vi "SParam Configure Measurement.vi"(8 "error in":errorcluster, 10 "Test Configuration":T2={"Action"=enum."Measure", "Power Level (dBm)"=0.0, "External Gain (dB)"=0.0, "Frequency Sweep"={"Start Frequency (Hz)"=4000000000.0, "Stop Frequency (Hz)"=26000000000.0, "Step Size (Hz)"=200.0}, "Type of Stimulus"=enum."CW", "Pulse Width (s)"=0.0, "PRI (s)"=0.0, "IF Bandwidth (Hz)"=0.0, "Average Mode"=enum."Per Sweep", "Number of Averages"=0, "SnP File Path"=path "", "Calibration File Path"=path ""} {"Frequency Sweep"."Step Size (Hz)" format="%#_6p"; "Frequency Sweep"."Stop Frequency (Hz)" format="%.3p"; "Frequency Sweep"."Start Frequency (Hz)" format="%.3p"}, 11 "S-Par Reference In":T1) -> (0 "error out":errorcluster, 3 "S-Par Reference Out":T1)   [LabVIEW 2023]
uses:
  <vilib>/niSPML/Typedefs/Session Handle.ctl
  <vilib>/niSPML/S-Par Reference.lvclass
  Controls/Test Config - SParam_VST.ctl
  <vilib>/niSPML/S-Parameter Measurements.lvlib
  <vilib>/niSPML/Configure Stimulus (CW).vi
  <vilib>/niSPML/Configure Stimulus (Pulsed CW).vi
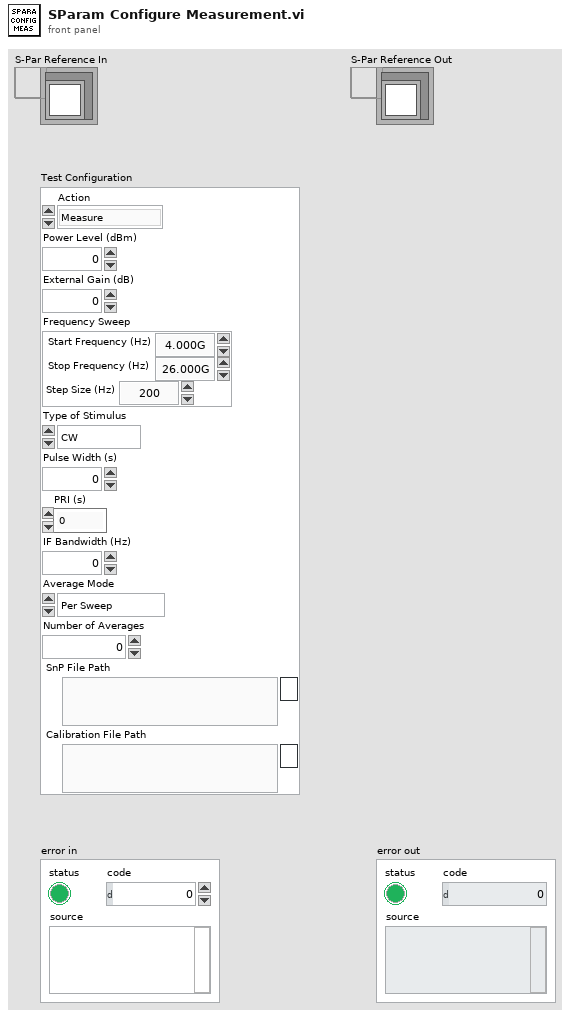
[diagram p1: front panel]
types:
  T1 = typedef "S-Parameter Measurements.lvlib/S-Par Reference.lvclass/Session Handle.ctl" = refnum<data-value>
  T2 = typedef "Test Config - SParam_VST.ctl" = cluster{"Action":enum32{"Calibrate", "Measure"}, "Power Level (dBm)":dbl, "External Gain (dB)":dbl, "Frequency Sweep":cluster{"Start Frequency (Hz)":dbl, "Stop Frequency (Hz)":dbl, "Step Size (Hz)":dbl}, "Type of Stimulus":enum16{"CW", "Pulsed CW"}, "Pulse Width (s)":dbl, "PRI (s)":dbl, "IF Bandwidth (Hz)":dbl, "Average Mode":enum16{"Per Sweep", "Per Point"}, "Number of Averages":i32, "SnP File Path":path, "Calibration File Path":path}
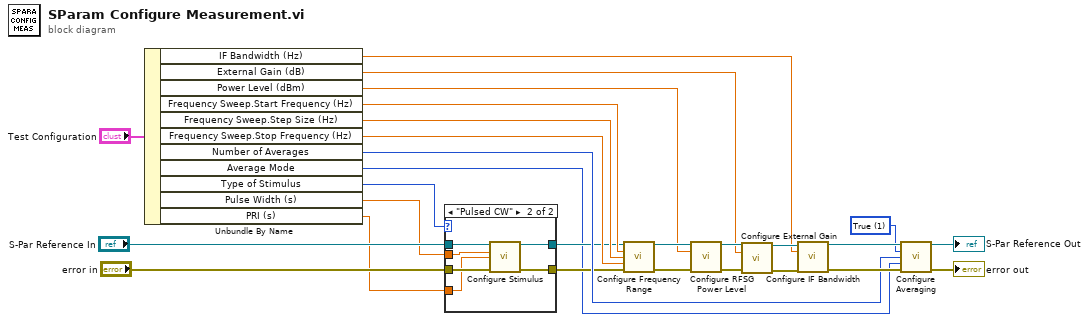
[diagram p0: block diagram]
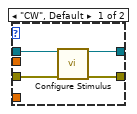
[diagram p2: hidden frame]
diagram:
  w19 = 1 items=["False", "True"] ("Averaging Enabled")
  n1 = Unbundle By Name("Test Configuration") -> ("IF Bandwidth (Hz)"=w12:dbl, "External Gain (dB)"=w13:dbl, "Power Level (dBm)"=w14:dbl, "Frequency Sweep.Start Frequency (Hz)"=w17:dbl, "Frequency Sweep.Step Size (Hz)"=w16:dbl, "Frequency Sweep.Stop Frequency (Hz)"=w15:dbl, "Number of Averages"=w11:i32, "Average Mode"=w1:enum16{"Per Sweep", "Per Point"}, "Type of Stimulus"=w8:enum16{"CW", "Pulsed CW"}, "Pulse Width (s)"=w3:dbl, "PRI (s)"=w2:dbl)
  n2 = case shown="\"Pulsed CW\"" w8 {
    tunnel: "S-Par Reference In" -> [w31 w37]
    tunnel: [w30 w36] -> w6
    tunnel: "error in" -> [w29 w35]
    tunnel: [w28 w34] -> w4
    tunnel: w3 -> [_ w33]
    tunnel: w2 -> [_ w32]
    frame "CW", Default {
      n3 = call-poly <vilib>:"Configure Stimulus.vi"("S-Par Reference In"=w31, "error in"=w29) -> ("S-Par Reference Out"=w30:T1, "error out"=w28:errorcluster)  [unwired: 12 in]
    }
    frame "Pulsed CW" {
      n4 = call-poly <vilib>:"Configure Stimulus.vi"("S-Par Reference In"=w37, "Pulse Width (s)"=w33, "PRI (s)"=w32, "error in"=w35) -> ("S-Par Reference Out"=w36:T1, "error out"=w34:errorcluster)  [unwired: 10 in]
    }
  }
  n5 = call <vilib>:"Configure Frequency Range.vi"("S-Par Reference In"=w6, "Start Frequency (Hz)"=w17, "Frequency Step (Hz)"=w16, "Stop Frequency (Hz)"=w15, "error in"=w4) -> ("S-Par Reference Out"=w21:T1, "error out"=w20:errorcluster)  [unwired: 9 in]
  n6 = call <vilib>:"Configure RFSG Power Level.vi"("S-Par Reference In"=w21, "Power Level (dBm)"=w14, "error in"=w20) -> ("S-Par Reference Out"=w27:T1, "error out"=w26:errorcluster)  [unwired: 11 in]
  n7 = call <vilib>:"Configure External Gain.vi"("S-Par Reference In"=w27, "External Gain (dB)"=w13, "error in"=w26) -> ("S-Par Reference Out"=w25:T1, "error out"=w24:errorcluster)  [unwired: 11 in]
  n8 = call <vilib>:"Configure IF Bandwidth.vi"("S-Par Reference In"=w25, "IF Bandwidth (Hz)"=w12, "error in"=w24) -> ("S-Par Reference Out"=w23:T1, "error out"=w22:errorcluster)  [unwired: 11 in]
  n9 = call <vilib>:"Configure Averaging.vi"("S-Par Reference In"=w23, "Averaging Enabled"=w19, "Averaging Count"=w11, "Averaging Type"=w1, "error in"=w22) -> ("S-Par Reference Out"=→"S-Par Reference Out":T1, "error out"=→"error out":errorcluster)  [unwired: 9 in]
